vi "Inspect VI.vi"(8 "error in (no error)":errorcluster, 11 "VI Path":path=path "C:/dev/SoL/sol-word-search/Scorer (2024Q1)/Scorer/Naughty VI Test.vi") -> (0 "error out":errorcluster, 2 "Issues":string[](array[string]))   [LabVIEW 2024, in "Wordle Scorer.lvlib"]
uses:
  Wordle Scorer.lvlib
  <vilib>/Utility/traverseref.llb/VI Scripting - Traverse.lvlib
  <vilib>/Utility/traverseref.llb/TRef TravTarget.ctl
  <vilib>/_script/All Supported PropertiesOrMethods TypeDefs/ASPM_UniqueIDStringDatanameShortnameLongname.ctl
panel:
  out "Properties":T1[](array[typedef])
  out "Style":string
  out "SubVIs":path[](array[path])
  out "Functions":string[](array[string])
  out "Unhandled Classes":string[](array[string])
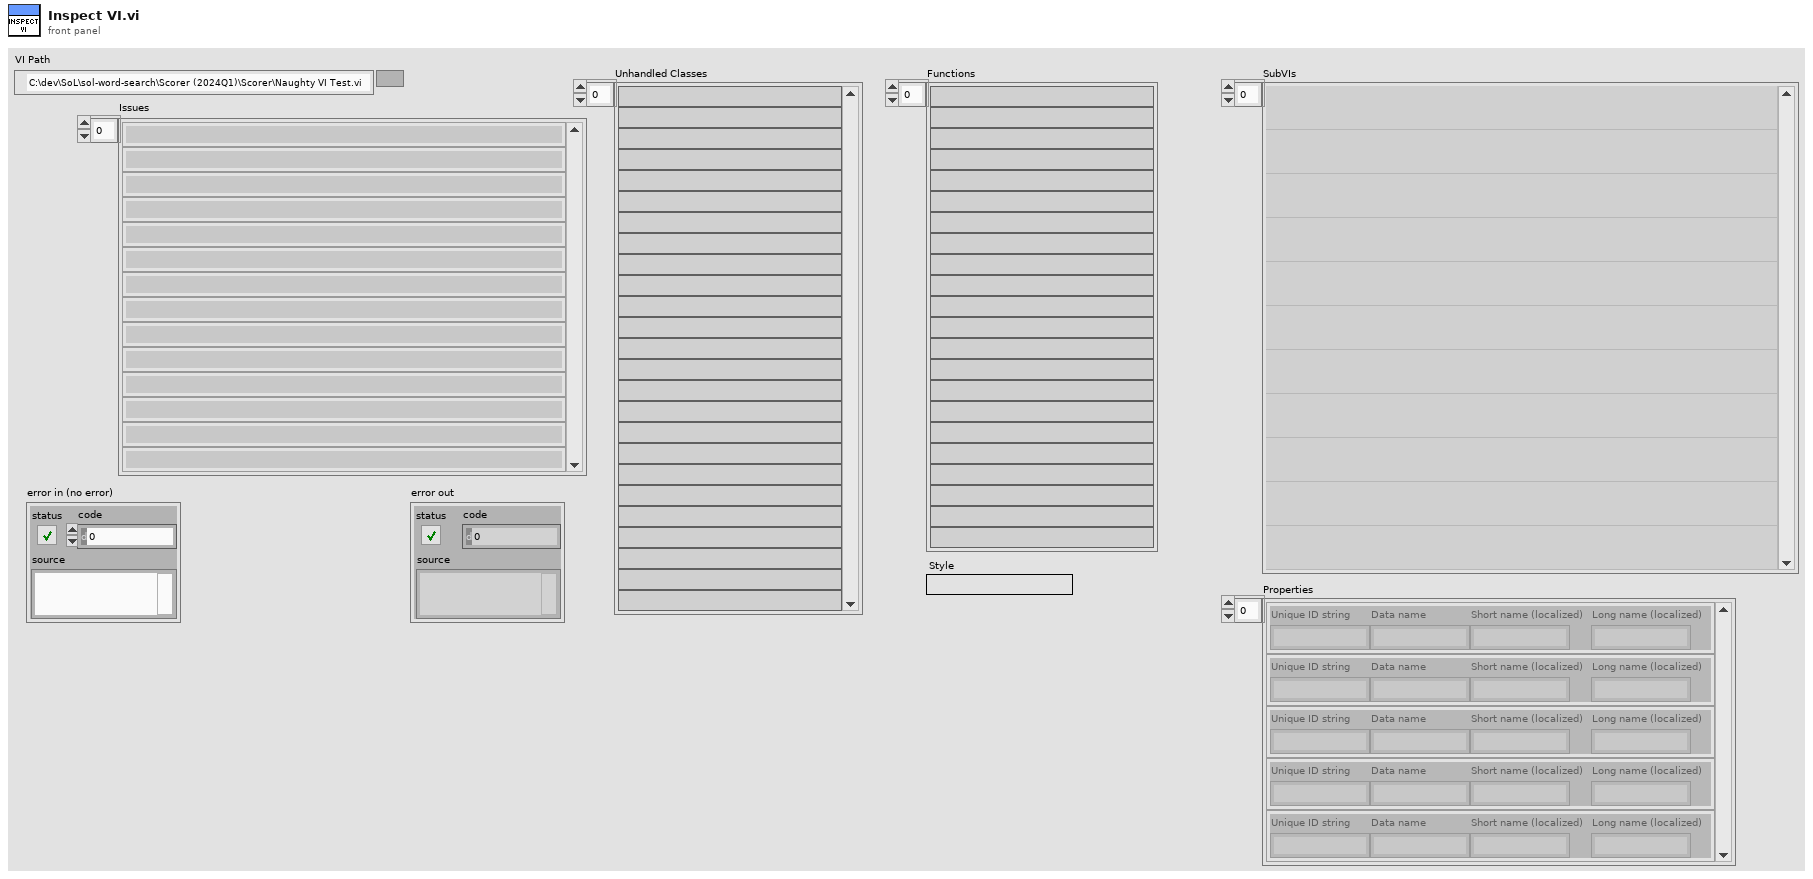
[diagram p1: front panel]
types:
  T1 = typedef "ASPM_UniqueIDStringDatanameShortnameLongname.ctl" = cluster{"Unique ID string":string, "Data name":string, "Short name (localized)":string, "Long name (localized)":string}
  T2 = typedef "TRef TravTarget.ctl" = enum16{"FP", "BD", "Other"}
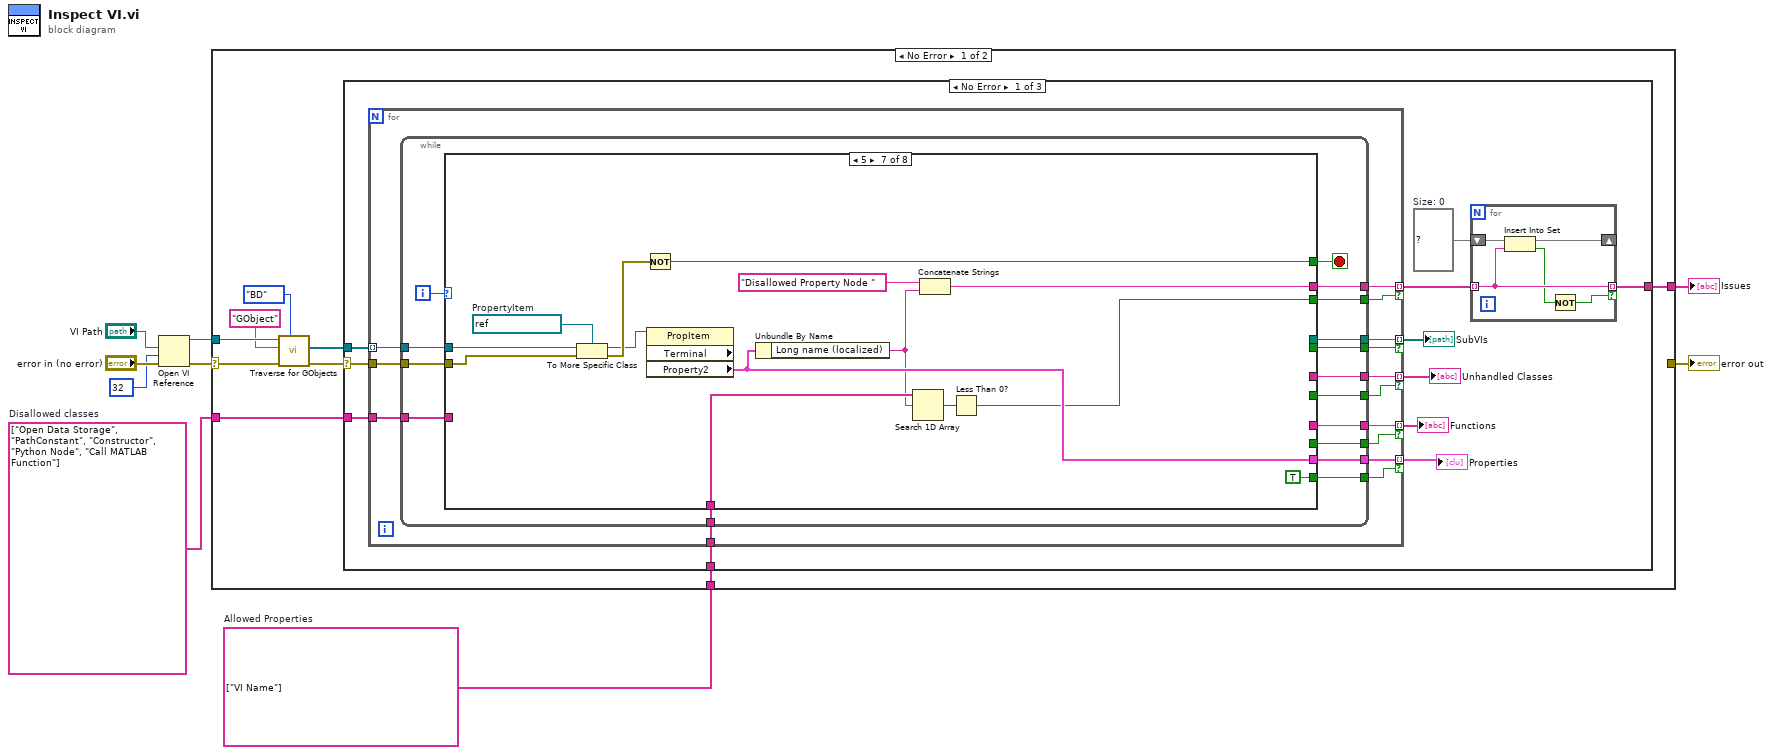
[diagram p0: block diagram]
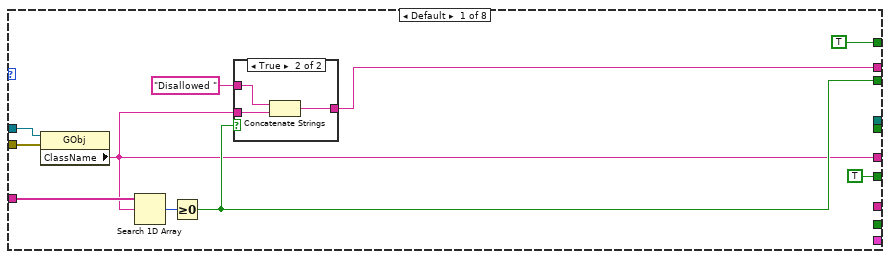
[diagram p2: hidden frame]
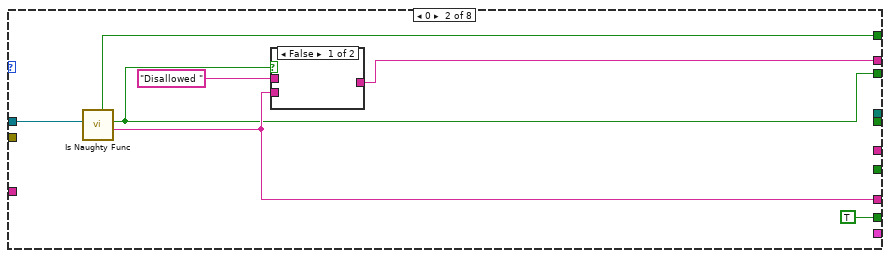
[diagram p4: hidden frame]
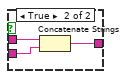
[diagram p5: hidden frame]
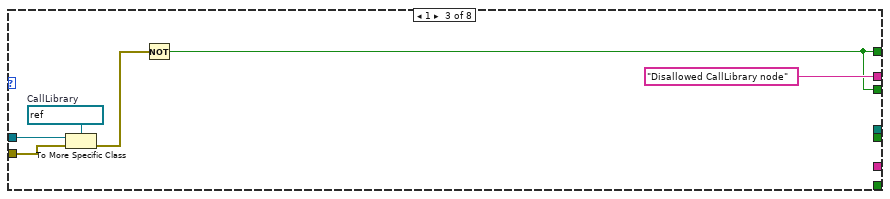
[diagram p6: hidden frame]
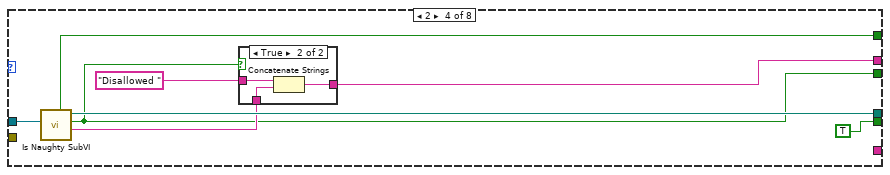
[diagram p7: hidden frame]
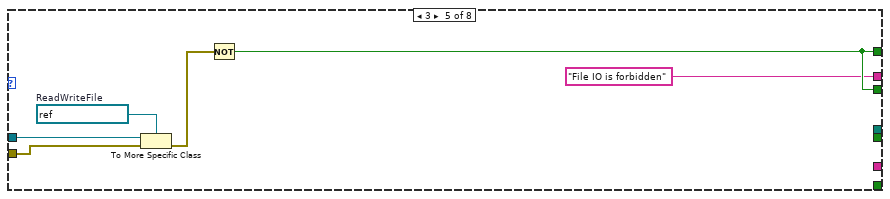
[diagram p9: hidden frame]
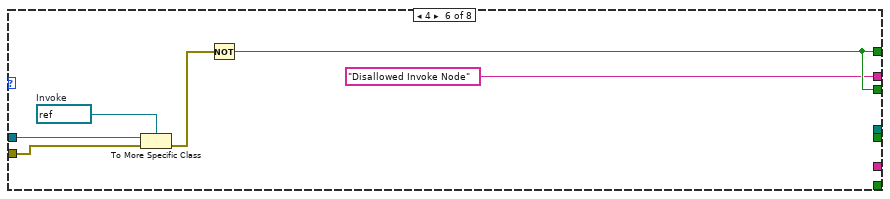
[diagram p10: hidden frame]
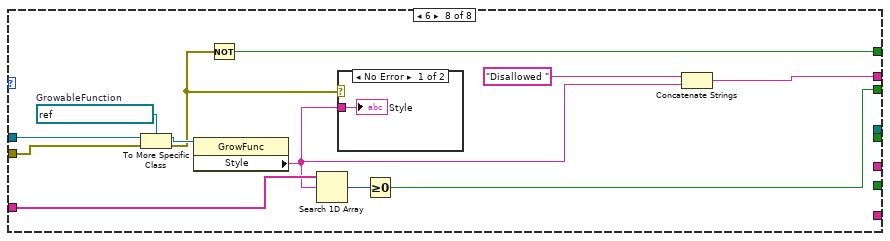
[diagram p11: hidden frame]
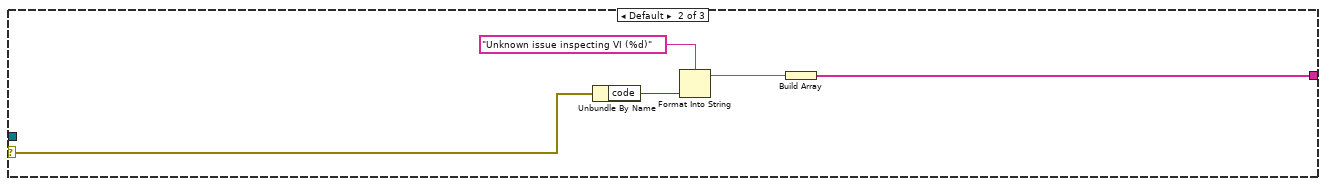
[diagram p13: hidden frame]
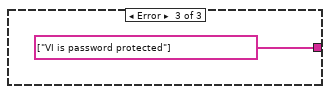
[diagram p14: hidden frame]
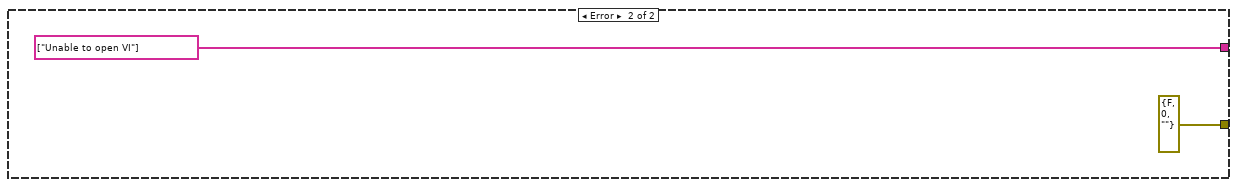
[diagram p15: hidden frame]
diagram:
  w1 = string[] ["VI Name"]  # Allowed Properties
  w2 = string[] ["Open Data Storage", "PathConstant", "Constructor", "Python Node", "Call MATLAB Function"]  # Disallowed classes
  n1 = Open VI Reference(vi path="VI Path", options=32, error in (no error)="error in (no error)") -> (vi reference=w5:refnum<vi>, error out=w6:errorcluster)  [unwired: 3 in]
  n2 = case shown="No Error" w6 {
    selector: w6 -> [w17 _]
    tunnel: w5 -> [w18 _]
    tunnel: [w12 string[] ["Unable to open VI"]] -> w4
    tunnel: [_ errorcluster {"status"=FALSE, "code"=0, "source"=""} ("error constant")] -> w3
    tunnel: w2 -> [w11 _]
    tunnel: w1 -> [w10 _]
    frame No Error {
      n3 = call <vilib>:"Traverse for GObjects.vi"("Traverse Target"=TRef_TravTarget."BD", "error in (no error)"=w17, "Class Name"="GObject", "VI Refnum"=w18) -> ("error out"=w13:errorcluster, "References"=w14:refnum<vi>[])  [unwired: 4 in, 2 out]
      n4 = case shown="No Error" w13 {
        selector: w13 -> [w28 w144 _]
        tunnel: w14 -> [w29 _ _]
        tunnel: [w21 w145 string[] ["VI is password protected"]] -> w12
        tunnel: w11 -> [w24 _ _]
        tunnel: w10 -> [w19 _ _]
        frame No Error {
          w22 = set{string} {}  # Size: 0
          n5 = for {
            tunnel: w29 -> [w48] mode=indexing
            tunnel: w28 -> [w47]
            tunnel: [w46] -> w27 mode=indexing if=w45
            tunnel: [w44] -> w26 mode=indexing if=w43
            tunnel: [w42] -> w23 mode=indexing if=w41
            tunnel: [w40] -> w25 mode=indexing if=w39
            tunnel: w24 -> [w38]
            tunnel: [w37] -> w20 mode=indexing if=w36
            tunnel: w19 -> [w35]
            n6 = while {
              tunnel: w48 -> [w62]
              tunnel: w47 -> [w61]
              tunnel: [w60] -> w46
              tunnel: [w59] -> w45
              tunnel: [w58] -> w44
              tunnel: [w57] -> w43
              tunnel: [w56] -> w42
              tunnel: [w55] -> w41
              tunnel: [w54] -> w40
              tunnel: [w53] -> w39
              tunnel: w38 -> [w52]
              tunnel: [w51] -> w37
              tunnel: [w50] -> w36
              tunnel: w35 -> [w49]
              i -> [w64]
              stop <- w63 stop-if-true
              n7 = case shown="5" w64 {
                tunnel: [TRUE w78 w88 w99 w106 w112 w124 w135] -> w63
                tunnel: w62 -> [w72 w83 w93 w94 w110 w116 w130 w142]
                tunnel: w61 -> [w73 _ w92 _ w109 w115 w129 w141]
                tunnel: [w66 _ _ _ _ _ _ _] -> w60
                tunnel: [TRUE _ _ _ _ _ _ _] -> w59
                tunnel: [_ w81 _ _ _ _ _ _] -> w58
                tunnel: [_ TRUE _ _ _ _ _ _] -> w57
                tunnel: [w65 w80 "Disallowed CallLibrary node" w96 "File IO is forbidden" "Disallowed Invoke Node" w119 w132] -> w56
                tunnel: [w68 w79 w88 w95 w106 w112 w120 w134] -> w55
                tunnel: [_ _ _ w101 _ _ _ _] -> w54
                tunnel: [_ _ _ TRUE _ _ _ _] -> w53
                tunnel: w52 -> [w70 _ _ _ _ _ _ w137]
                tunnel: [_ _ _ _ _ _ w123 _] -> w51
                tunnel: [_ _ _ _ _ _ TRUE _] -> w50
                tunnel: w49 -> [_ _ _ _ _ _ w122 _]
                frame Default {
                  n8 = property class="GObj"(reference=w72, error in=w73) -> ("ClassName"=w66:string)  [unwired: 2 out]
                  n9 = Search 1D Array(1D array=w70, element=w66) -> (index of element=w69:i32)  [unwired: 1 in]
                  n10 = Greater Or Equal To 0?(x=w69) -> (x >= 0?=w68:bool)
                  n11 = case shown="True" w68 {
                    tunnel: "Disallowed " -> [_ w77]
                    tunnel: w66 -> [_ w76]
                    tunnel: [_ w75] -> w65
                    frame False {
                    }
                    frame True {
                      n12 = Concatenate Strings(w77, w76) -> (w75:string)
                    }
                  }
                }
                frame 0 {
                  n13 = call "Is Naughty Func.vi"("GObj Refnum"=w83) -> ("Function"=w81:string, "Naughty Function"=w79:bool, "Is Func"=w78:bool)  [unwired: 8 in]
                  n14 = case shown="False" w79 {
                    tunnel: "Disallowed " -> [_ w87]
                    tunnel: w81 -> [_ w86]
                    tunnel: [_ w85] -> w80
                    frame False {
                    }
                    frame True {
                      n15 = Concatenate Strings(w87, w86) -> (w85:string)
                    }
                  }
                }
                frame 1 {
                  w91 = refnum<vi> refnum  # CallLibrary
                  n16 = To More Specific Class(target class=w91, reference=w93, error in=w92) -> (error out=w90:errorcluster)  [unwired: 1 out]
                  n17 = Not(x=w90) -> (.not. x?=w88:bool)
                }
                frame 2 {
                  n18 = call "Is Naughty SubVI.vi"("GObj Refnum"=w94) -> ("SubVI"=w97:string, "Naughty SubVI"=w95:bool, "VIPath"=w101:path, "Is SubVI"=w99:bool)  [unwired: 7 in]
                  n19 = case shown="True" w95 {
                    tunnel: "Disallowed " -> [_ w104]
                    tunnel: w97 -> [_ w103]
                    tunnel: [_ w102] -> w96
                    frame False {
                    }
                    frame True {
                      n20 = Concatenate Strings(w104, w103) -> (w102:string)
                    }
                  }
                }
                frame 3 {
                  w108 = refnum<vi> refnum  # ReadWriteFile
                  n21 = To More Specific Class(target class=w108, reference=w110, error in=w109) -> (error out=w107:errorcluster)  [unwired: 1 out]
                  n22 = Not(x=w107) -> (.not. x?=w106:bool)
                }
                frame 4 {
                  w114 = refnum<vi> refnum  # Invoke
                  n23 = To More Specific Class(target class=w114, reference=w116, error in=w115) -> (error out=w113:errorcluster)  [unwired: 1 out]
                  n24 = Not(x=w113) -> (.not. x?=w112:bool)
                }
                frame 5 {
                  w128 = refnum<vi> refnum  # PropertyItem
                  n25 = To More Specific Class(target class=w128, reference=w130, error in=w129) -> (specific class reference=w117:refnum<vi>, error out=w127:errorcluster)
                  n26 = Not(x=w127) -> (.not. x?=w124:bool)
                  n27 = property class="PropItem" props=["Terminal", "Property2"](reference=w117) -> ("Property2"=w123:T1)  [unwired: 1 in, 3 out]
                  n28 = Unbundle By Name(w123) -> ("Long name (localized)"=w118:string)
                  n29 = Search 1D Array(1D array=w122, element=w118) -> (index of element=w121:i32)  [unwired: 1 in]
                  n30 = Concatenate Strings("Disallowed Property Node ", w118) -> (w119:string)
                  n31 = Less Than 0?(x=w121) -> (x < 0?=w120:bool)
                }
                frame 6 {
                  w140 = refnum<vi> refnum  # GrowableFunction
                  n32 = To More Specific Class(target class=w140, reference=w142, error in=w141) -> (specific class reference=w138:refnum<vi>, error out=w133:errorcluster)
                  n33 = property class="GrowFunc"(reference=w138) -> ("Style"=w131:string)  [unwired: 1 in, 2 out]
                  n34 = Not(x=w133) -> (.not. x?=w135:bool)
                  n35 = Search 1D Array(1D array=w137, element=w131) -> (index of element=w136:i32)  [unwired: 1 in]
                  n36 = case shown="No Error" w133 {
                    tunnel: w131 -> [w143 _]
                    frame No Error {
                      "Style" <- w143
                    }
                    frame Error {
                    }
                  }
                  n37 = Greater Or Equal To 0?(x=w136) -> (x >= 0?=w134:bool)
                  n38 = Concatenate Strings("Disallowed ", w131) -> (w132:string)
                }
              }
            }
          }
          "Unhandled Classes" <- w27
          "Functions" <- w26
          "SubVIs" <- w25
          "Properties" <- w20
          n39 = for {
            tunnel: w23 -> [w32] mode=indexing
            shift-right: [w33] -> _
            shift-left: w22 -> [w34]
            tunnel: [w32] -> w21 mode=indexing if=w30
            n40 = Insert Into Set(10:w32, 11:w34) -> (2:w31:bool, 3:w33:set{string})
            n41 = Not(x=w31) -> (.not. x?=w30:bool)
          }
        }
        frame Default {
          n42 = Unbundle By Name(w144) -> ("code"=w147:i32)
          n43 = Format Into String(format string="Unknown issue inspecting VI (%d)", w147) -> (resulting string=w146:string)  [unwired: 2 in, 1 out]
          n44 = Build Array(w146) -> (w145:string[])
        }
        frame Error {
        }
      }
    }
    frame Error {
    }
  }
  "error out" <- w3
  "Issues" <- w4
